vi "pcfs_check_notifier_for_exit.vi"(8 "error in (no error)":errorcluster, 11 "pcfs in":refnum<class "pcfs.lvclass">) -> (0 "error out":errorcluster, 2 "exit?":bool, 3 "pcfs out":refnum<class "pcfs.lvclass">)   [LabVIEW 2015, in "pcfs.lvclass"]
uses:
  pcfs.lvclass
  pcfs.lvclass/pcfs.ctl
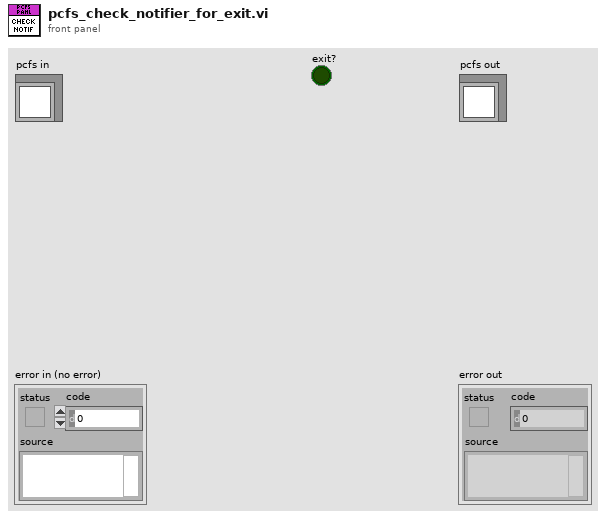
[diagram p1: front panel]
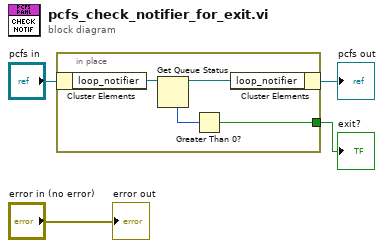
[diagram p0: block diagram]
diagram:
  n1 = in-place {
    in-place-border: [w5] -> w1
    n2 = in-place-cluster #1("pcfs in") -> ("loop_notifier"=w8:refnum<queue>)
    n3 = Get Queue Status(queue=w8) -> (queue out=w6:refnum<queue>, # elements in queue=w7:i32)  [unwired: 2 in, 6 out]
    n4 = Greater Than 0?(x=w7) -> (x > 0?=w5:bool)
    n5 = in-place-cluster #1("loop_notifier"=w6) -> (→"pcfs out":refnum<class "pcfs.lvclass">)
  }
  "exit?" <- w1
  "error out" <- "error in (no error)"
